vi "push_to_grab_image.vi"(8 "Boolean 2":bool, 10 "picture":picture) -> ()   [LabVIEW 2015]
uses:
  Control_drona_19.11.2016/video_global.vi
panel:
  in  "Boolean":bool
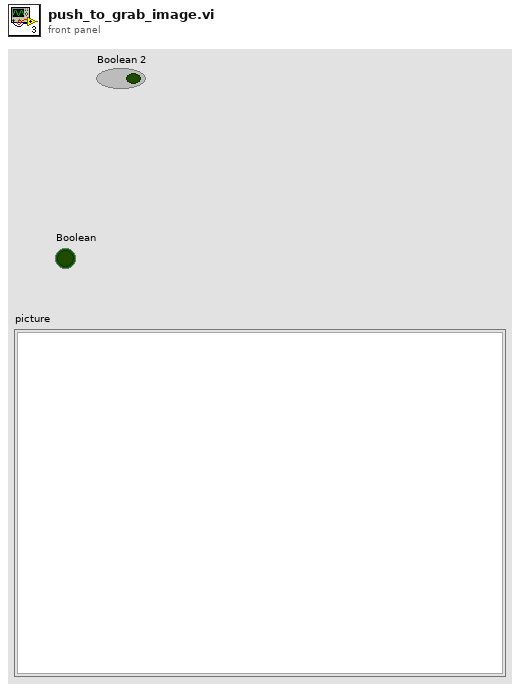
[diagram p1: front panel]
types:
  T1 = typedef "imagedata.ctl" = cluster{"image type":i32, "image depth":i32, "image":u8[], "mask":u8[], "colors":u32[], "Rectangle":cluster{"left":i16, "top":i16, "right":i16, "bottom":i16}}
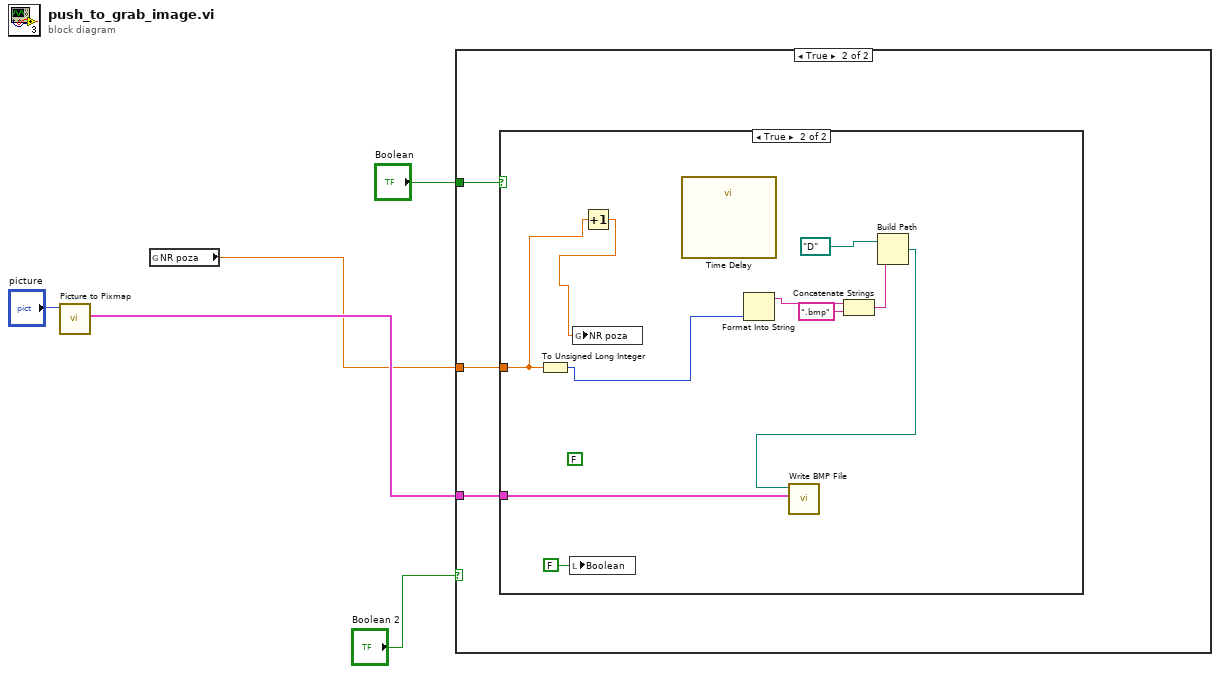
[diagram p0: block diagram]
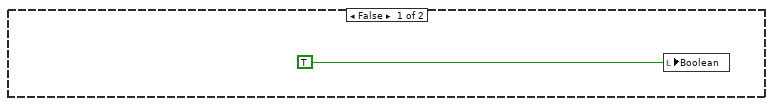
[diagram p2: hidden frame]
diagram:
  n1 = call <vilib>:"Picture to Pixmap.vi"("picture"="picture") -> ("image data"=w5:T1)  [unwired: 9 in, 1 out]
  n2 = global read "video_global.vi" "NR poza"() -> (w1:dbl)
  n3 = case shown="True" "Boolean 2" {
    tunnel: "Boolean" -> [_ w9]
    tunnel: w5 -> [_ w8]
    tunnel: w1 -> [_ w7]
    frame False {
      n4 = local write "Boolean"(TRUE) -> ()
    }
    frame True {
      n5 = case shown="True" w9 {
        tunnel: w8 -> [_ w13]
        tunnel: w7 -> [_ w11]
        frame False {
        }
        frame True {
          (unwired) FALSE ("Compress? (N)")
          n6 = To Unsigned Long Integer(number=w11) -> (unsigned 32bit integer=w12:u32)
          n7 = local write "Boolean"(FALSE) -> ()
          n8 = Increment(x=w11) -> (x+1=w10:dbl)
          n9 = global write "video_global.vi" "NR poza"(w10) -> ()
          n10 = call "Time Delay"() -> ()  [unwired: 11 in, 1 out]
          n11 = Format Into String(w12) -> (resulting string=w17:string)  [unwired: 3 in, 1 out]
          n12 = Concatenate Strings(w17, ".bmp" ("string")) -> (w15:string)
          n13 = Build Path(base path=path "D:/", name or relative path=w15) -> (appended path=w14:path)
          n14 = call <vilib>:"Write BMP File.vi"("image data"=w13, "path to BMP file"=w14) -> ()  [unwired: 8 in, 2 out]
        }
      }
    }
  }
